vi "ManualTemperature.vi"() -> (0 "Humidity [%] out":dbl, 1 "Temperature [°C] out":dbl)   [LabVIEW 2019]
panel:
  in  "rel. Humidity [%]":dbl
  in  "OK Button":bool
  in  "Temperature [°C]":dbl
  # "Please enter \ntemperature & humidiy"
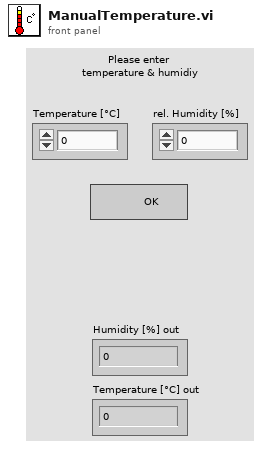
[diagram p1: front panel]
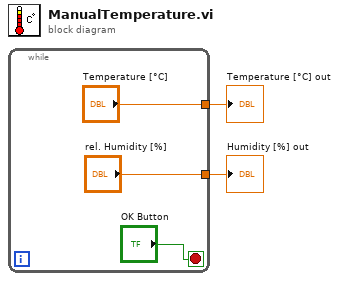
[diagram p0: block diagram]
diagram:
  n1 = while {
    tunnel: ["Temperature [°C]"] -> w2
    tunnel: ["rel. Humidity [%]"] -> w1
    stop <- "OK Button" stop-if-true
  }
  "Temperature [°C] out" <- w2
  "Humidity [%] out" <- w1
